vi "Refine Corner Locations.vi"(5 "Termination Criteria (Default: Default Criteria) in":refnum<class "Termination Criteria.lvclass">, 6 "Zero Zone Size (Default: -1 x -1)":T1={"Width"=-1, "Height"=-1}, 7 "Window Size (Default: 11 x 11)":T1={"Width"=11, "Height"=11}, 8 "error in (no error)":errorcluster, 10 "Points in":T2[](array[typedef]), 11 "Greyscale Image in":T3) -> (0 "error out":errorcluster, 2 "Points out":T2[](array[typedef]), 3 "Greyscale Image":T3)   [LabVIEW 2020, in "feature_detection.lvlib"]
doc: "Refine the Corner Locations in an image. This can be used to improve the precision of the points returned by the Find Chessboard Corners.vi."
uses:
  feature_detection.lvlib
  image/Greyscale Image.ctl
  common/Image Point (Float).ctl
  common/Termination Criteria/Termination Criteria.lvclass
  common/Window Size (Integer).ctl
  common/Termination Criteria/Termination Criteria.lvclass/Termination Criteria.ctl
  common/common.lvlib
  common/bin/gartoolkit_32-1.dll
  image/image.lvlib
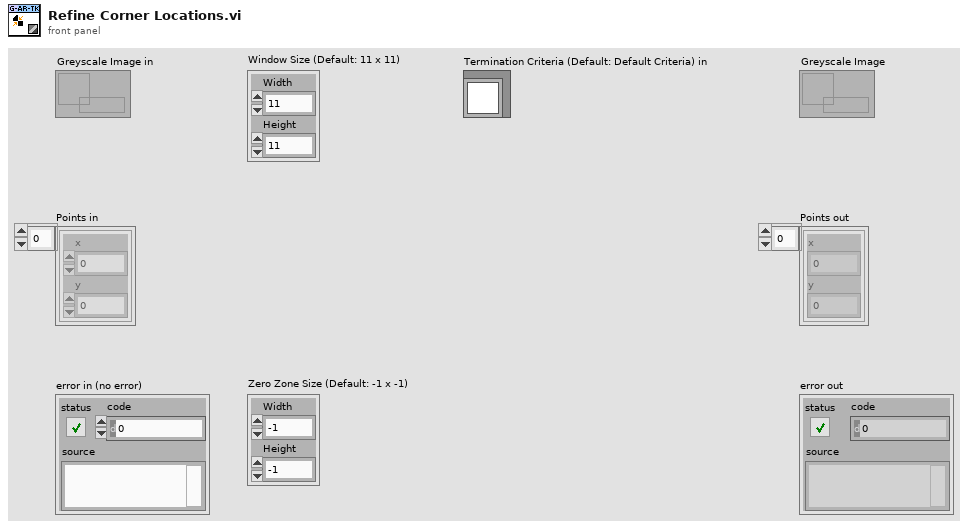
[diagram p1: front panel]
types:
  T1 = typedef "common.lvlib/Window Size (Integer).ctl" = cluster{"Width":i32, "Height":i32}
  T2 = typedef "common.lvlib/Image Point (Float).ctl" = cluster{"x":dbl, "y":dbl}
  T3 = typedef "image.lvlib/Greyscale Image.ctl" = refnum<data-value>
  T4 = typedef "common.lvlib/Termination Criteria.lvclass/Termination Criteria Values.ctl" = cluster{"Epsilon":dbl, "Iterations":i32}
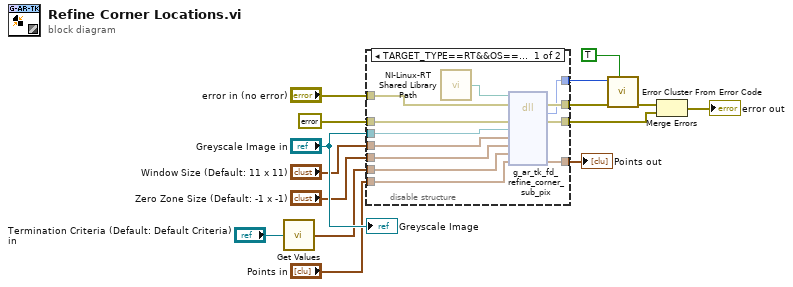
[diagram p0: block diagram]
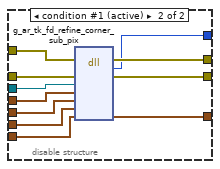
[diagram p2: hidden frame]
diagram:
  n1 = call "Get Values.vi"("Termination Criteria in"="Termination Criteria (Default: Default Criteria) in") -> ("Term Criteria"=w7:T4)
  n2 = disable-structure shown="TARGET_TYPE==RT&&OS==Linux" {
    disable-tunnel: "error in (no error)" -> [w26 w38]
    disable-tunnel: errorcluster {"status"=FALSE, "code"=0, "source"=""} ("error constant") -> [w25 w37]
    disable-tunnel: "Greyscale Image in" -> [w24 w36]
    disable-tunnel: "Window Size (Default: 11 x 11)" -> [w23 w35]
    disable-tunnel: "Zero Zone Size (Default: -1 x -1)" -> [w22 w34]
    disable-tunnel: w7 -> [w21 w33]
    disable-tunnel: "Points in" -> [w20 w32]
    disable-tunnel: [w19 w31] -> w5
    disable-tunnel: [w18 w30] -> w4
    disable-tunnel: [w17 w29] -> w3
    disable-tunnel: [w16 w28] -> w2
    frame condition #0 {
      n3 = call "NI-Linux-RT Shared Library Path.vi"() -> ("Path"=w27:path)
      n4 = dll-call lib="?" fn="g_ar_tk_fd_refine_corner_sub_pix" ("g_ar_toolkit.*.*:g_ar_tk_image_draw_line")(path in=w27, error in=w26, "error_cluster"=w25, "EDVR src"=w24, "Window Size"=w23, "Zero Zone"=w22, "Termination Criteria"=w21, "Points"=w20) -> (error out=w19:errorcluster, w18:i32, "error_cluster"=w17:errorcluster, "Points"=w16:T2[])  [unwired: 5 in, 1 out]
    }
    frame condition #1 (active) {
      n5 = dll-call lib="C:/serenial/lib/g-augmented-reality-toolkit/LabVIEW/common/bin/gartoolkit_*-1.*" fn="g_ar_tk_fd_refine_corner_sub_pix" ("g_ar_toolkit.*.*:g_ar_tk_image_draw_line")(error in=w38, "error_cluster"=w37, "EDVR src"=w36, "Window Size"=w35, "Zero Zone"=w34, "Termination Criteria"=w33, "Points"=w32) -> (error out=w31:errorcluster, w30:i32, "error_cluster"=w29:errorcluster, "Points"=w28:T2[])  [unwired: 6 in, 1 out]
    }
  }
  "Points out" <- w2
  n6 = call <vilib>:"Error Cluster From Error Code.vi"("show call chain? (False)"=TRUE, "error in (no error)"=w5, "error code (0)"=w4) -> ("error out"=w15:errorcluster)  [unwired: 6 in]
  n7 = Merge Errors(w15, w3) -> (→"error out":errorcluster)
  "Greyscale Image" <- "Greyscale Image in"
